vi "RW Mods.vi"(0 "RSI Modules in":T1[](array[typedef]) {"Module Config Data"."Config Block Data Refs"."Data Reference" format="%.0x"; "CDOutput Data"."BD Refs"."Data Reference" format="%.0x"; "CDInput Data"."BD Refs"."Data Reference" format="%.0x"; "VS ref" format="%.0x"}, 1 "R/W Case":T14, 5 "Input Mod Size Idxs":T12, 7 "Output modules":i32[](array[numeric]), 9 "MixedIO Mod Size Idxs":T12, 11 "error in (no error)":errorcluster, 12 "Async in":T13) -> (4 "RSI Modules out":T1[](array[typedef]) {"Module Config Data"."Config Block Data Refs"."Data Reference" format="%.0x"; "CDOutput Data"."BD Refs"."Data Reference" format="%.0x"; "CDInput Data"."BD Refs"."Data Reference" format="%.0x"; "VS ref" format="%.0x"}, 14 "Async out":T13, 15 "error out":errorcluster)   [LabVIEW 2019, in "SEECD Engine.lvlib"]
uses:
  SEECD Engine.lvlib
  Type Defs/RSI Module Data.ctl
  <vilib>/NI VeriStand/Custom Device API/Custom Device Item Ref.ctl
  Type Defs/Open Module IOVs.ctl
  Modules.lvlibp/RSI Module/RSI Module.lvclass
  Modules.lvlibp/RSI Module/Module Models.ctl
  Modules.lvlibp/RSI Module/Channel Type.ctl
  Type Defs/Input Data.ctl
  <vilib>/NI VeriStand/Custom Device API/Block Data Reference.ctl
  <vilib>/NI VeriStand/Custom Device API/Data Reference.ctl
  Type Defs/Output Data.ctl
  Type Defs/Module Config Data.ctl
  Type Defs/Mixed IO.ctl
  Type Defs/RW Case.ctl
  Type Defs/Async Data.ctl
  Type Defs/Async Status.ctl
  Type Defs/Async State.ctl
  Type Defs/Async Command.ctl
  Type Defs/Mod Size Indexes.ctl
  Read Input Modules at Indexes.vi
  Read Mixed Modules at Indexes.vi
  <vilib>/NI VeriStand/Custom Device API/NI VeriStand - Get Channel Values by Block Data Reference.vi
  Scanned Write - Module.vi
  Read Input Module.vi
  Read Mixed Module.vi
  <vilib>/NI VeriStand/Custom Device API/NI VeriStand - Set Channel Values by Block Data Reference.vi
  Scanned Read - Input Module.vi
  Scanned Read - Mixed Module.vi
  <vilib>/NI VeriStand/Custom Device API/Global Data Refs.vi
  Launch Local Reconfig.vi
  <vilib>/NI VeriStand/Custom Device API/Custom Device API.lvlib
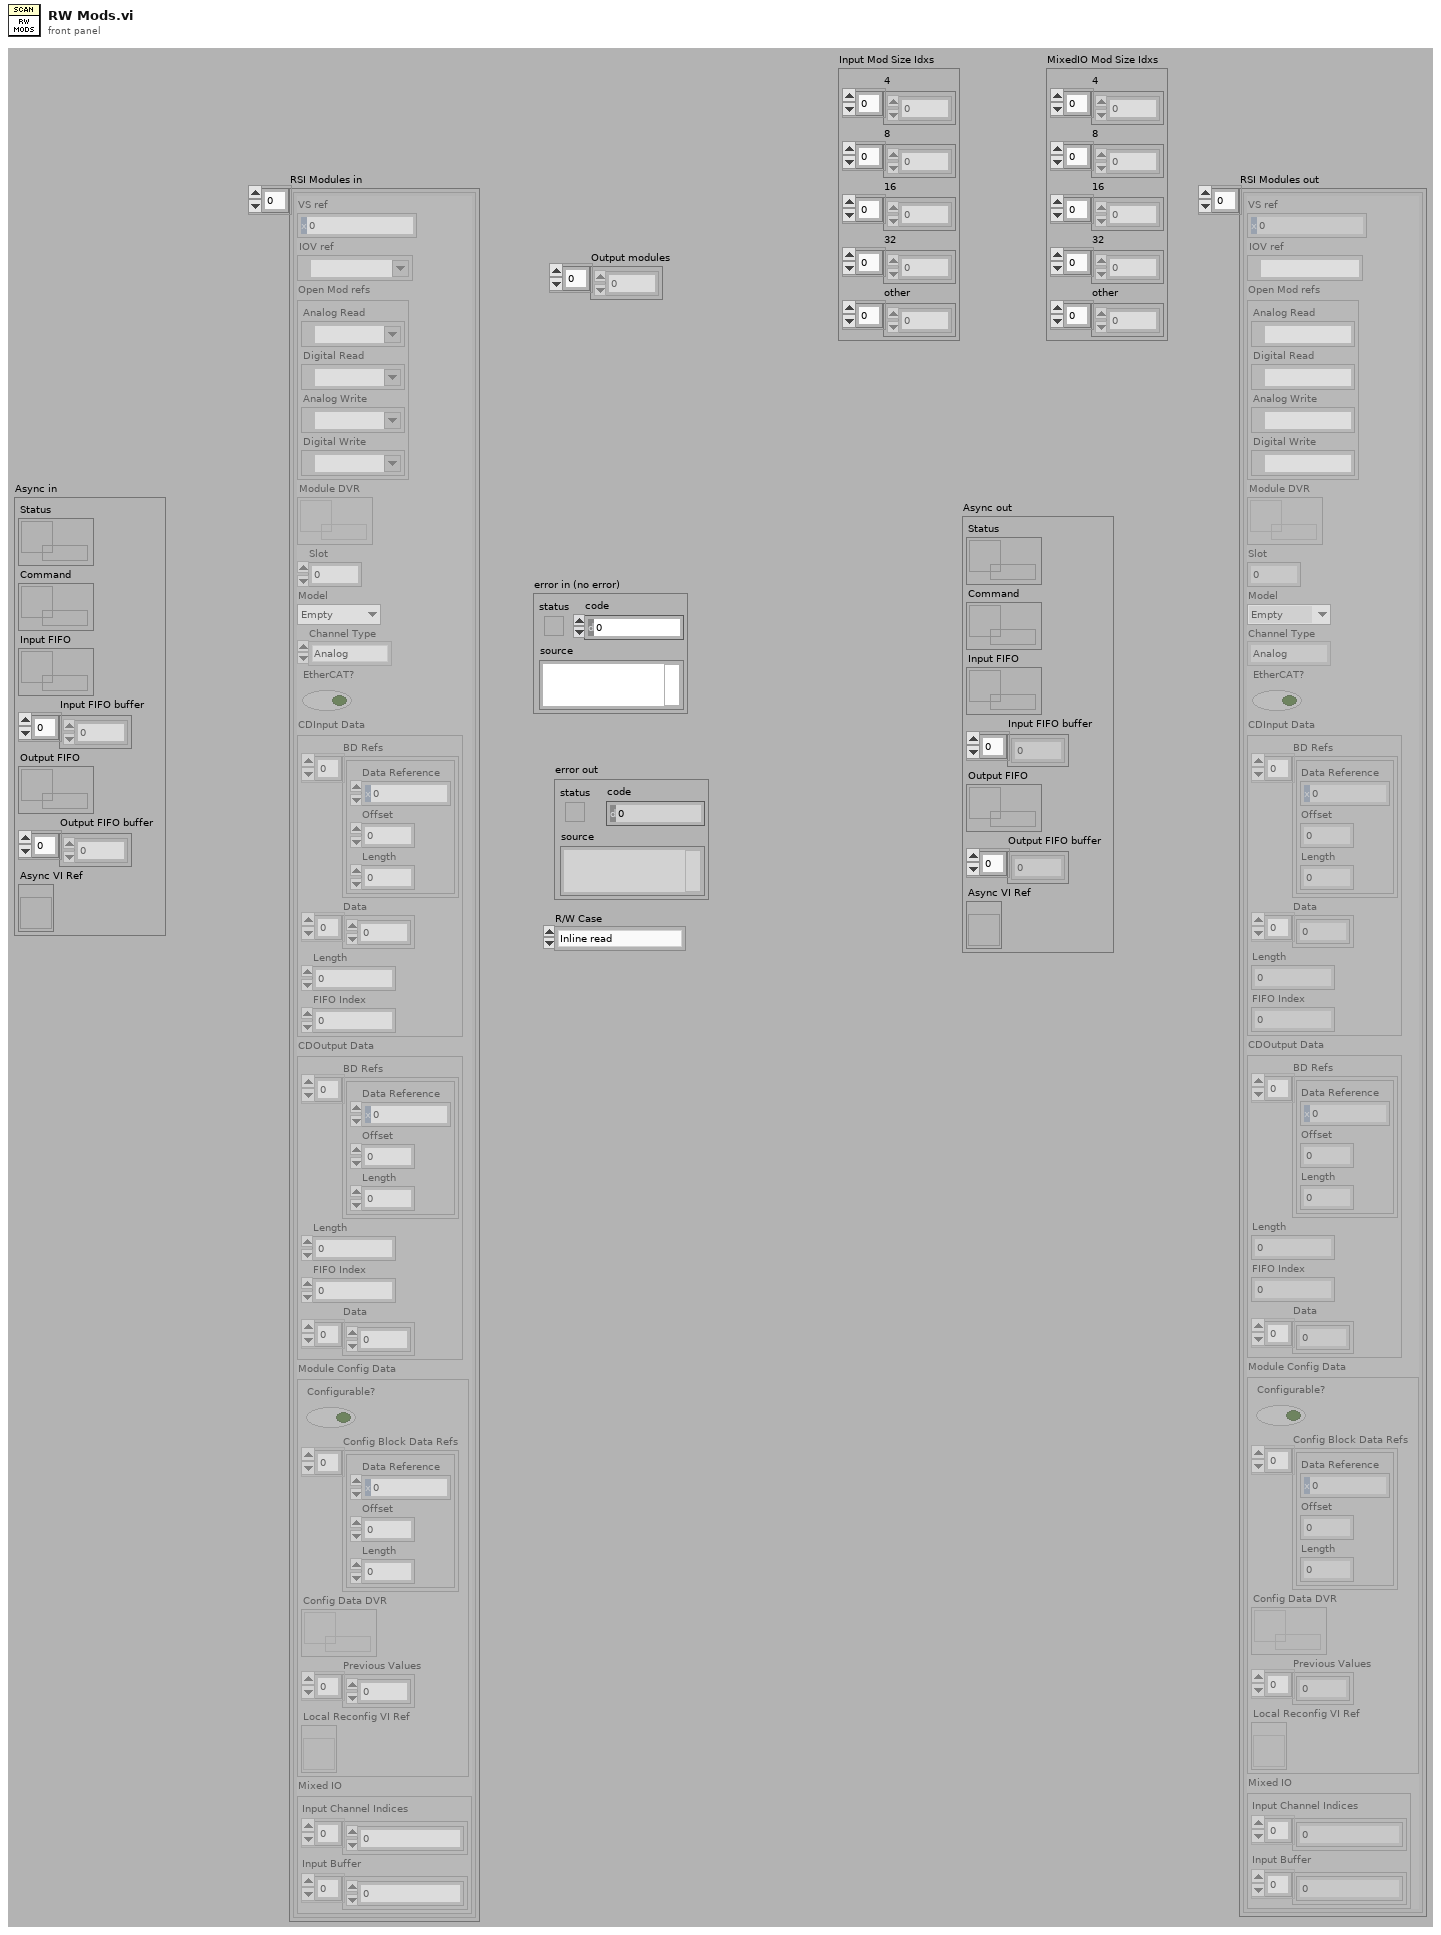
[diagram p1: front panel]
types:
  T1 = typedef "SEECD Engine.lvlib/RSI Module Data.ctl" = cluster{"VS ref":T2, "IOV ref":refnum<k21>, "Open Mod refs":T3, "Module DVR":refnum<data-value>, "Slot":u32, "Model":T4, "Channel Type":T5, "EtherCAT?":bool, "CDInput Data":T6, "CDOutput Data":T9, "Module Config Data":T10, "Mixed IO":T11}
  T2 = typedef "Custom Device API.lvlib/Custom Device Item Ref.ctl" = u64
  T3 = typedef "SEECD Engine.lvlib/Open Module IOVs.ctl" = cluster{"Analog Read":refnum<k21>, "Digital Read":refnum<k21>, "Analog Write":refnum<k21>, "Digital Write":refnum<k21>}
  T4 = typedef "Modules.lvlibp/RSI Module.lvclass/Module Models.ctl" = enum16{"Empty", "NI 9201", "NI 9203", "NI 9205", "NI 9206", "NI 9207", "NI 9208", "NI 9209", "NI 9210", "NI 9211", "NI 9212", "NI 9213", "NI 9214", "NI 9215", "NI 9216", "NI 9217", "NI 9219", "NI 9220", "NI 9221", "NI 9222", "NI 9223", "NI 9224", "NI 9225", "NI 9226", "NI 9227", "NI 9228", "NI 9229", "NI 9233", "NI 9234", "NI 9235", "NI 9236", "NI 9237", "NI 9239", "NI 9242", "NI 9244", "NI 9253", "NI 9263", "NI 9264", "NI 9265", "NI 9266", "NI 9269", "NI 9344", "NI 9350", "NI 9375", "NI 9401", "NI 9402", "NI 9403", "NI 9411", "NI 9421", "NI 9422", "NI 9423", "NI 9425", "NI 9426", "NI 9435", "NI 9436", "NI 9437", "NI 9472", "NI 9474", "NI 9475", "NI 9476", "NI 9477", "NI 9478", "NI 9481", "NI 9482", "NI 9485"}
  T5 = typedef "Modules.lvlibp/RSI Module.lvclass/Channel Type.ctl" = enum16{"Analog", "Digital"}
  T6 = typedef "SEECD Engine.lvlib/Input Data.ctl" = cluster{"BD Refs":T7[], "Data":dbl[], "Length":i32, "FIFO Index":i32}
  T7 = typedef "Custom Device API.lvlib/Block Data Reference.ctl" = cluster{"Data Reference":T8, "Offset":u64, "Length":u64}
  T8 = typedef "Custom Device API.lvlib/Data Reference.ctl" = i32
  T9 = typedef "SEECD Engine.lvlib/Output Data.ctl" = cluster{"BD Refs":T7[], "Length":i32, "FIFO Index":i32, "Data":dbl[]}
  T10 = typedef "SEECD Engine.lvlib/Module Config Data.ctl" = cluster{"Configurable?":bool, "Config Block Data Refs":T7[], "Config Data DVR":refnum<data-value>, "Previous Values":dbl[], "Local Reconfig VI Ref":refnum<vi>}
  T11 = typedef "SEECD Engine.lvlib/Mixed IO.ctl" = cluster{"Input Channel Indices":i32[], "Input Buffer":dbl[]}
  T12 = typedef "SEECD Engine.lvlib/Mod Size Indexes.ctl" = cluster{"4":i32[], "8":i32[], "16":i32[], "32":i32[], "other":i32[]}
  T13 = typedef "SEECD Engine.lvlib/Async Data.ctl" = cluster{"Status":refnum<queue>, "Command":refnum<queue>, "Input FIFO":refnum<k33>, "Input FIFO buffer":dbl[], "Output FIFO":refnum<k33>, "Output FIFO buffer":dbl[], "Async VI Ref":refnum<vi>}
  T14 = typedef "SEECD Engine.lvlib/RW Case.ctl" = enum16{"Inline read", "Inline write", "Async - Inline loop read", "Async - Inline loop write", "Async loop (read/write)"}
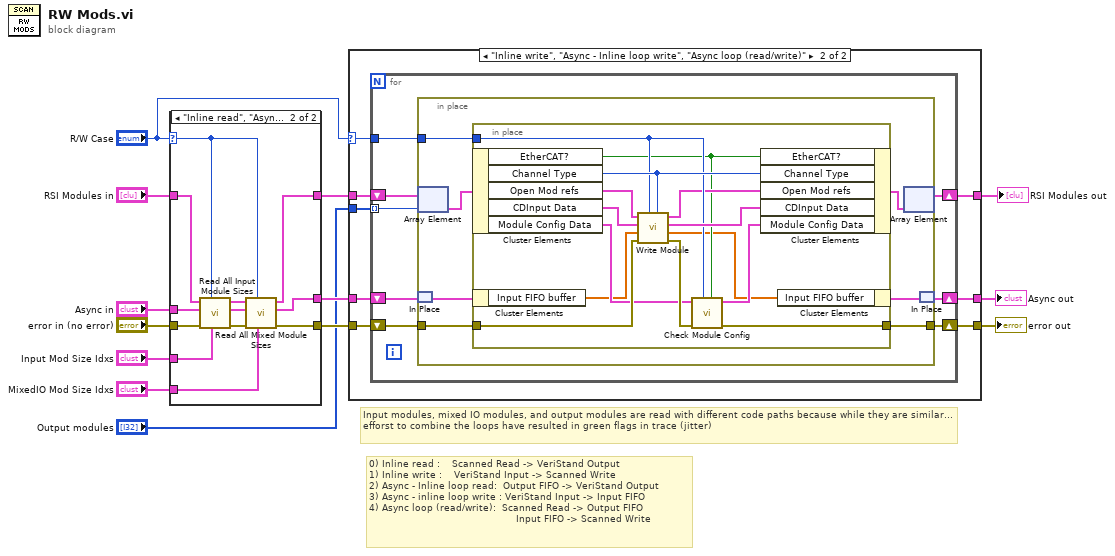
[diagram p0: block diagram]
diagram:
  # "Input modules, mixed IO modules, and output modules are read with different code paths because while they are similar... efforst to combine the loops have resulted in green flags in trace (jitter)"
  # "0) Inline read\t:\t\t\t\tScanned Read -> VeriStand Output\n1) Inline write\t:\t\t\t\tVeriStand Input -> Scanned Write\n2) Async - Inline loop read:\t\tOutput FIFO -> VeriStand Output\n3) Async - inline loop write\t: VeriStand Input -> Input FIFO\n4) Async loop (read/write):\t\tScanned Read -> Output FIFO\n\t\t\t\t\t                                            Input FIFO -> Scanned Write"
  n1 = case shown="\"Inline read\", \"Async - Inline loop read\", \"Async loop (read/write)\"" "R/W Case" {
    selector: "R/W Case" -> [_ w17]
    tunnel: "RSI Modules in" -> [w14 w22]
    tunnel: "error in (no error)" -> [w15 w28]
    tunnel: "Async in" -> [w16 w23]
    tunnel: [w15 w25] -> w10
    tunnel: [w16 w26] -> w9
    tunnel: [w14 w24] -> w5
    tunnel: "Input Mod Size Idxs" -> [_ w21]
    tunnel: "MixedIO Mod Size Idxs" -> [_ w18]
    frame Default {
    }
    frame "Inline read", "Async - Inline loop read", "Async loop (read/write)" {
      n2 = call "Read All Input Module Sizes.vi"("Input Mod Size Idxs"=w21, "R/W Case"=w17, "error in (no error)"=w28, "Async in"=w23, "RSI Modules in"=w22) -> ("error out"=w27:errorcluster, "Async out"=w20:T13, "RSI Modules out"=w19:T1[])  [unwired: 4 in]
      n3 = call "Read All Mixed Module Sizes.vi"("MixedIO Mod Size Idxs"=w18, "R/W Case"=w17, "error in (no error)"=w27, "Async in"=w20, "RSI Modules in"=w19) -> ("error out"=w25:errorcluster, "Async out"=w26:T13, "RSI Modules out"=w24:T1[])  [unwired: 4 in]
    }
  }
  n4 = case shown="\"Inline write\", \"Async - Inline loop write\", \"Async loop (read/write)\"" "R/W Case" {
    selector: "R/W Case" -> [_ w37]
    tunnel: w10 -> [w31 w39]
    tunnel: w5 -> [w29 w33]
    tunnel: w9 -> [w30 w38]
    tunnel: [w31 w36] -> w6
    tunnel: [w30 w35] -> w7
    tunnel: [w29 w34] -> w4
    tunnel: "Output modules" -> [_ w32]
    frame Default {
    }
    frame "Inline write", "Async - Inline loop write", "Async loop (read/write)" {
      n5 = for {
        shift-right: [w43] -> w36
        shift-left: w39 -> [w46]
        shift-right: [w45] -> w34
        shift-left: w33 -> [w47]
        tunnel: w37 -> [w44]
        shift-right: [w41] -> w35
        shift-left: w38 -> [w42]
        tunnel: w32 -> [w40] mode=indexing
        n6 = in-place {
          in-place-border: w46 -> [w53]
          in-place-border: w44 -> [w51]
          in-place-border: [w50] -> w43
          n7 = in-place-array #1(w47, w40) -> (w54:T1)
          n8 = in-place-match #2(w42) -> (w49:T13)
          n9 = in-place {
            in-place-border: w53 -> [w68]
            in-place-border: w51 -> [w64]
            in-place-border: [w55] -> w50
            n10 = in-place-cluster #3(w54) -> ("EtherCAT?"=w59:bool, "Channel Type"=w65:T5, "Open Mod refs"=w56:T3, "CDInput Data"=w67:T6, "Module Config Data"=w61:T10)
            n11 = in-place-cluster #4(w49) -> ("Input FIFO buffer"=w58:dbl[])
            n12 = call "Write Module.vi"("Channel Type"=w65, "R/W Case"=w64, "error in (no error)"=w68, "Input FIFO buffer in"=w58, "Input Data in"=w67, "IOV ref in"=w56) -> ("error out"=w63:errorcluster, "Input FIFO buffer out"=w57:dbl[], "Input Data out"=w66:T6, "IOV ref out"=w62:T3)  [unwired: 2 in]
            n13 = call "Check Module Config.vi"("EtherCAT?"=w59, "R/W Case"=w64, "error in (no error)"=w63, "Module Config Data in"=w61) -> ("error out"=w55:errorcluster, "Module Config Data out"=w60:T10)  [unwired: 6 in]
            n14 = in-place-cluster #3("EtherCAT?"=w59, "Channel Type"=w65, "Open Mod refs"=w62, "CDInput Data"=w66, "Module Config Data"=w60) -> (w52:T1)
            n15 = in-place-cluster #4("Input FIFO buffer"=w57) -> (w48:T13)
          }
          n16 = in-place-array #1(w52) -> (w45:T1[])  [unwired: 1 out]
          n17 = in-place-match #2(w48) -> (w41:T13)
        }
      }
    }
  }
  "error out" <- w6
  "Async out" <- w7
  "RSI Modules out" <- w4
